vi "抓邊.vi"(0 "Image In":T1, 1 "Process":T7(ring), 2 "Optimized Mode":bool, 3 "Direction":T4(ring), 5 "ROI":T2, 9 "Gap":i32=10 min=1 max=300, 11 "error In":errorcluster, 12 "Edge Options":T5={"Edge Polarity"=0, "Kernel Size"=3, "Width"=3, "Minimum Edge Strength"=10.0, "Interpolation Type"=enum."Bilinear Fixed", "Data Processing Method"=enum."Average"} {"Edge Polarity" items=["All Edges", "Rising Edges", "Falling Edges"]; "Minimum Edge Strength" format="%.2f"; "Width" step=2; "Kernel Size" step=2}, 13 "Point Diameter (5)":u32=5 min=3 max=1000) -> (4 "Image Out":T1, 6 "Line Profile":T3(graph), 10 "Gradient Information":dbl[][](graph), 14 "Line Data":cluster{"X":sgl, "Y":sgl, "T":sgl}, 15 "error out":errorcluster)   [LabVIEW 2015]
uses:
  <vilib>/vision/Measure.llb/Edge Options.ctl
  <vilib>/vision/Measure.llb/Edge Polarity.ctl
  <vilib>/vision/Image Controls.llb/IMAQ Image.ctl
  <vilib>/vision/NI_Vision_Development_Module.lvlib
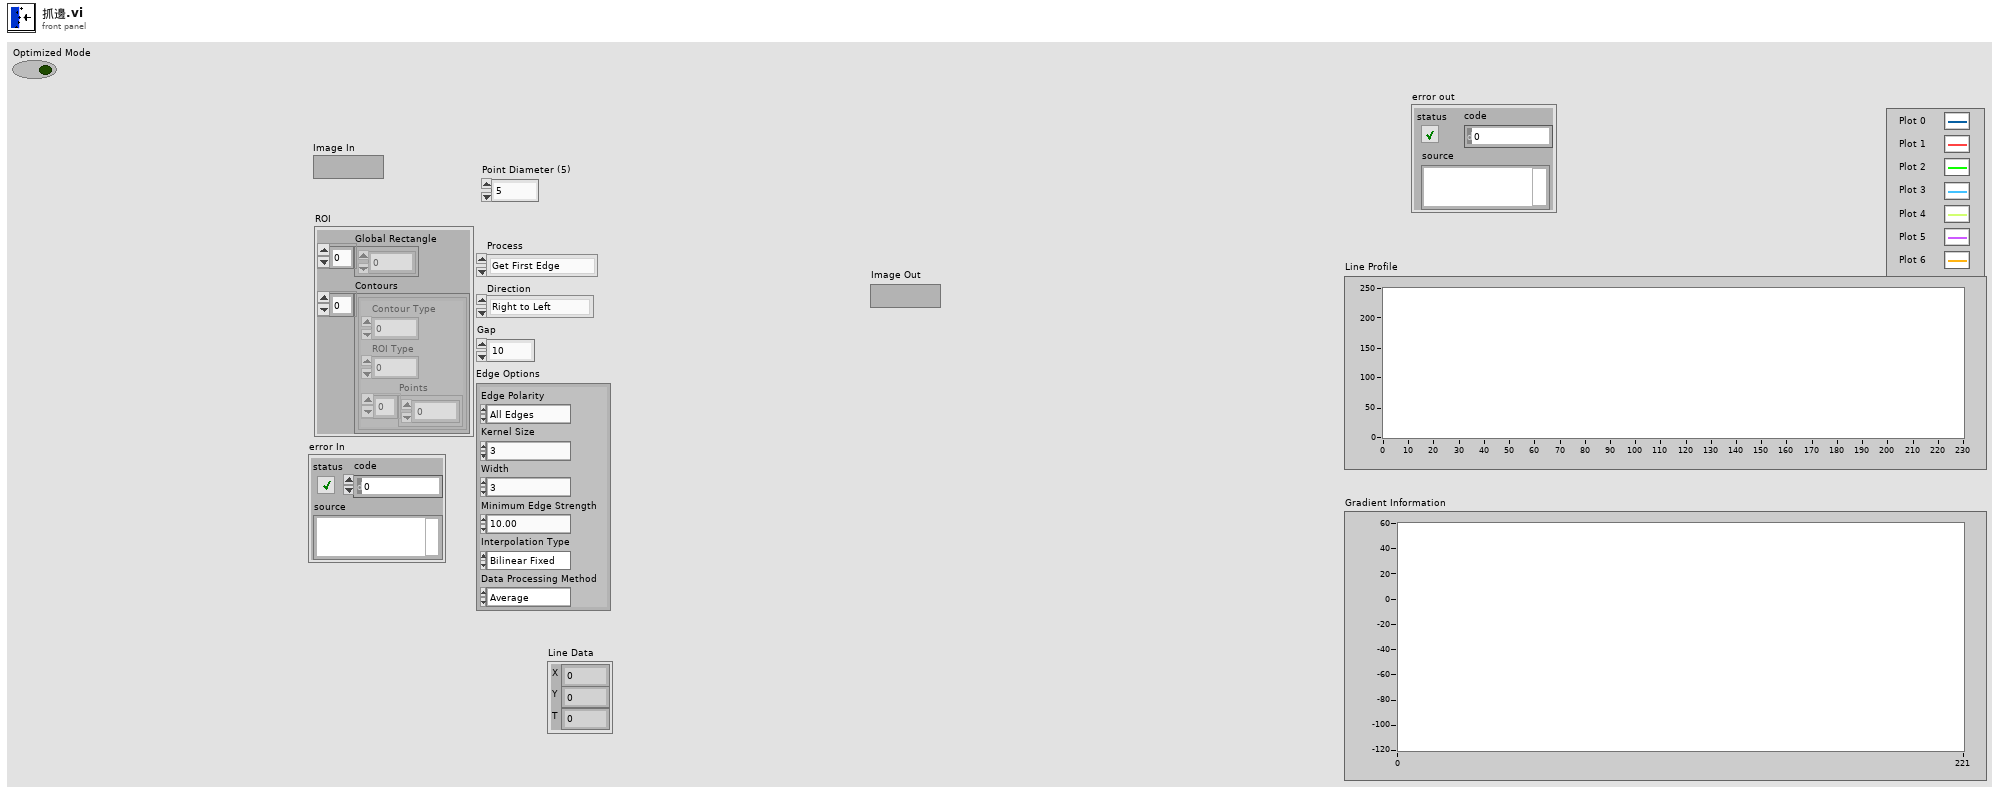
[diagram p1: front panel]
types:
  T1 = typedef "IMAQ Image.ctl" = refnum<image>
  T2 = cluster{"Global Rectangle":i32[], "Contours":cluster{"Contour Type":u32, "ROI Type":u32, "Points":i32[]}[]}
  T3 = cluster{"x0":sgl, "dx":sgl, "Pixels Line":sgl[]}[]
  T4 = enum16{"Right to Left", "Left  to Right", "Up to Down", "Down to Up"}
  T5 = typedef "Edge Options.ctl" = cluster{"Edge Polarity":T6, "Kernel Size":u32, "Width":u32, "Minimum Edge Strength":sgl, "Interpolation Type":enum32{"Zero Order", "Bilinear", "Quadratic", "Cubic", "Bilinear Fixed"}, "Data Processing Method":enum32{"Average", "Median"}}
  T6 = typedef "Edge Polarity.ctl" = u32
  T7 = enum16{"Get First Edge", "Get First + Last Edge", "Get All Edges", "Get Best Edge"}
  T8 = typedef "IMAQ Rectangle" = cluster{"Left":i32, "Top":i32, "Right":i32, "Bottom":i32, "Rotation":dbl}
  T9 = typedef "IMAQ Point" = cluster{"X":sgl, "Y":sgl}
  T10 = cluster{"Point 1":cluster{"x":dbl, "y":dbl}, "Point 2":cluster{"x":dbl, "y":dbl}}
  T11 = typedef "IMAQ Line" = cluster{"Start X":i32, "Start Y":i32, "End X":i32, "End Y":i32}
  T12 = typedef "ROI Descriptor" = cluster{"Global Rectangle":i32[], "Contours":cluster{"ID":enum32{"External", "Internal"}, "Type":u32, "Coordinates":i32[]}[]}
  T13 = typedef "Edge New.ctl" = cluster{"Location (Pixel)":cluster{"X":sgl, "Y":sgl}, "Location (Real-World)":cluster{"X":sgl, "Y":sgl}, "Distance (Pixel)":dbl, "Distance (Real-World)":dbl, "Strength":dbl, "Noise":dbl, "Rising?":bool}
  T14 = cluster{"Point 1":cluster{"X":sgl, "Y":sgl}, "Point 2":cluster{"X":sgl, "Y":sgl}}
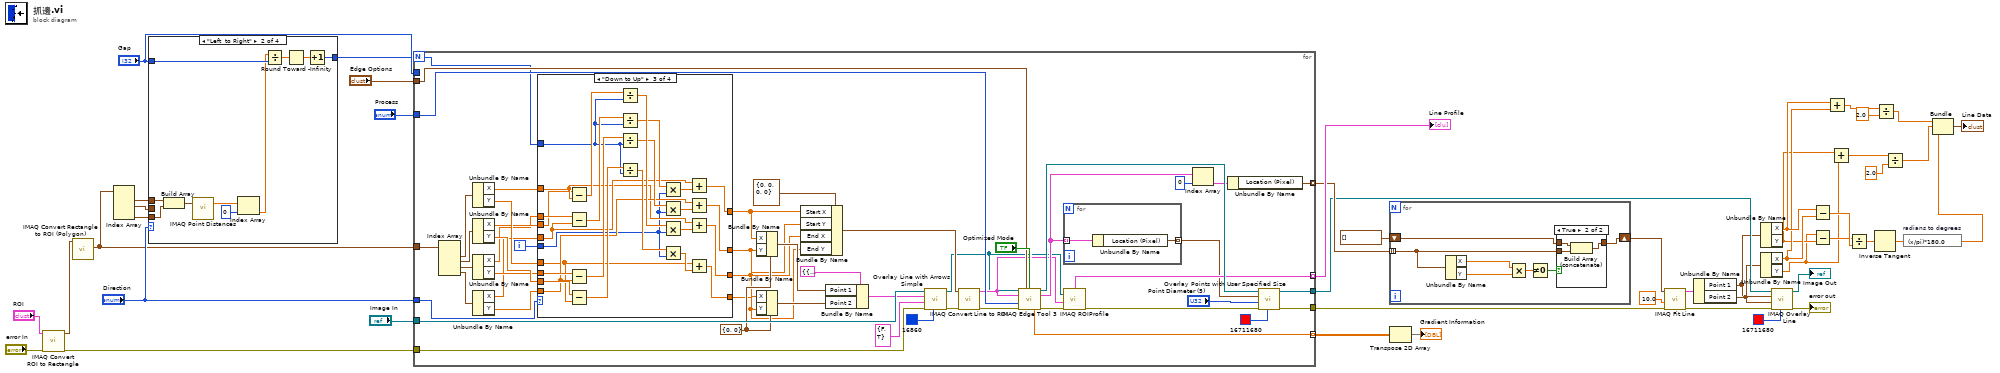
[diagram p0: block diagram]
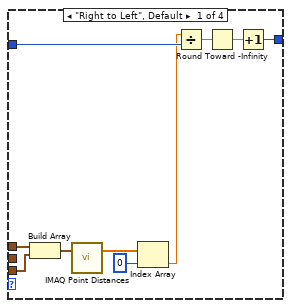
[diagram p2: hidden frame]
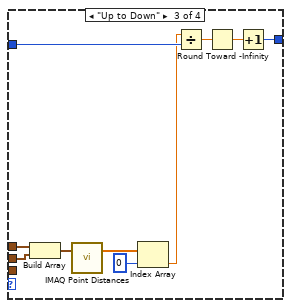
[diagram p3: hidden frame]
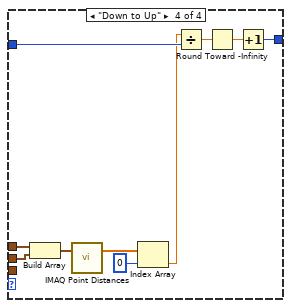
[diagram p4: hidden frame]
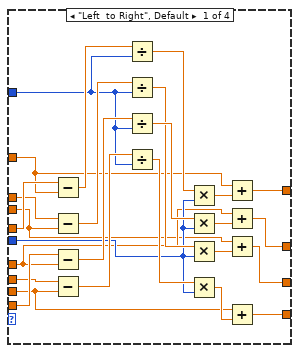
[diagram p6: hidden frame]
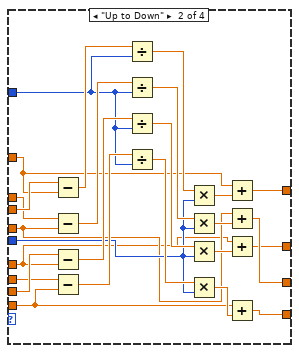
[diagram p7: hidden frame]
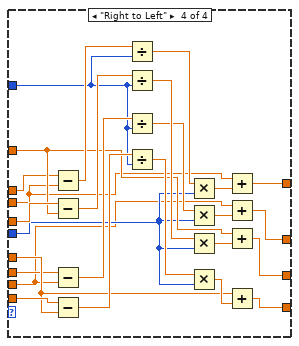
[diagram p8: hidden frame]
diagram:
  n1 = call "IMAQ Convert ROI to Rectangle"("error in (no error)"="error In", "ROI Descriptor"="ROI") -> ("error out"=w38:errorcluster, "Rectangle"=w26:T8)  [unwired: 7 in]
  n2 = call "IMAQ Convert Rectangle to ROI (Polygon)"("Rectangle"=w26) -> ("Rectangle Points"=w32:T9[])  [unwired: 7 in, 2 out]
  n3 = Index Array(array=w32) -> (element #1=w29:T9, element #2=w28:T9, element #4=w27:T9)  [unwired: 4 in, 1 out]
  n4 = case shown="\"Left  to Right\"" "Direction" {
    tunnel: "Gap" -> [w54 w64 w74 w84]
    tunnel: [w53 w63 w73 w83] -> w39
    tunnel: w29 -> [w50 w60 w72 w80]
    tunnel: w27 -> [w49 w59 _ _]
    tunnel: w28 -> [_ _ w68 w79]
    frame "Right to Left", Default {
      n5 = Build Array(w50, w49) -> (w52:T9[])
      n6 = call "IMAQ Point Distances"("Points"=w52) -> ("Distances"=w51:sgl[])  [unwired: 4 in, 1 out]
      n7 = Index Array(array=w51, index=0) -> (element=w47:sgl)
      n8 = Divide(x=w47, y=w54) -> (x/y=w55:sgl)
      n9 = Round Toward -Infinity(1:w55) -> (0:w56:sgl)
      n10 = Increment(x=w56) -> (x+1=w53:i32)
    }
    frame "Left  to Right" {
      n11 = Build Array(w60, w59) -> (w62:T9[])
      n12 = call "IMAQ Point Distances"("Points"=w62) -> ("Distances"=w61:sgl[])  [unwired: 4 in, 1 out]
      n13 = Index Array(array=w61, index=0) -> (element=w57:sgl)
      n14 = Divide(x=w57, y=w64) -> (x/y=w65:sgl)
      n15 = Round Toward -Infinity(1:w65) -> (0:w66:sgl)
      n16 = Increment(x=w66) -> (x+1=w63:i32)
    }
    frame "Up to Down" {
      n17 = Build Array(w72, w68) -> (w71:T9[])
      n18 = call "IMAQ Point Distances"("Points"=w71) -> ("Distances"=w70:sgl[])  [unwired: 4 in, 1 out]
      n19 = Index Array(array=w70, index=0) -> (element=w69:sgl)
      n20 = Divide(x=w69, y=w74) -> (x/y=w75:sgl)
      n21 = Round Toward -Infinity(1:w75) -> (0:w76:sgl)
      n22 = Increment(x=w76) -> (x+1=w73:i32)
    }
    frame "Down to Up" {
      n23 = Build Array(w80, w79) -> (w82:T9[])
      n24 = call "IMAQ Point Distances"("Points"=w82) -> ("Distances"=w81:sgl[])  [unwired: 4 in, 1 out]
      n25 = Index Array(array=w81, index=0) -> (element=w78:sgl)
      n26 = Divide(x=w78, y=w84) -> (x/y=w85:sgl)
      n27 = Round Toward -Infinity(1:w85) -> (0:w86:sgl)
      n28 = Increment(x=w86) -> (x+1=w83:i32)
    }
  }
  n29 = for {
    N: w39 -> [w124]
    tunnel: "Direction" -> [w122]
    tunnel: [w133] -> w35
    tunnel: "Image In" -> [w123]
    tunnel: w38 -> [w120]
    tunnel: [w132] -> w33
    tunnel: "Process" -> [w134]
    tunnel: "Edge Options" -> [w131]
    tunnel: [w130] -> w37 mode=indexing
    tunnel: [w129] -> w40 mode=indexing
    tunnel: [w128] -> w36 mode=indexing
    tunnel: "Gap" -> [_]
    tunnel: w32 -> [w119]
    i -> [w88]
    w116 = cluster{"X":i32, "Y":i32} {"X"=0, "Y"=0} ("Start Point")
    n30 = Index Array(array=w119) -> (element #1=w100:T9, element #2=w99:T9, element #3=w98:T9, element #4=w97:T9)  [unwired: 4 in]
    n31 = Unbundle By Name(w100) -> ("X"=w96:sgl, "Y"=w95:sgl)
    n32 = Unbundle By Name(w99) -> ("X"=w94:sgl, "Y"=w93:sgl)
    n33 = Unbundle By Name(w98) -> ("X"=w92:sgl, "Y"=w91:sgl)
    n34 = Unbundle By Name(w97) -> ("X"=w90:sgl, "Y"=w89:sgl)
    n35 = case shown="\"Down to Up\"" w122 {
      tunnel: [w149 w168 w194 w219] -> w108
      tunnel: [w144 w167 w193 w220] -> w105
      tunnel: [w147 w165 w191 w217] -> w107
      tunnel: [w143 w166 w192 w218] -> w106
      tunnel: w90 -> [w162 w173 w199 w229]
      tunnel: w96 -> [w140 w175 w198 w228]
      tunnel: w124 -> [w153 w177 w204 w230]
      tunnel: w88 -> [w152 w178 w195 w227]
      tunnel: w89 -> [w159 w169 w201 w224]
      tunnel: w95 -> [w142 w171 w200 w223]
      tunnel: w92 -> [w156 w174 w197 w226]
      tunnel: w94 -> [w141 w176 w196 w225]
      tunnel: w91 -> [w151 w170 w202 w222]
      tunnel: w93 -> [w139 w172 w203 w221]
      frame "Left  to Right", Default {
        n36 = Subtract(x=w162, y=w140) -> (x-y=w163:sgl)
        n37 = Subtract(x=w156, y=w141) -> (x-y=w158:sgl)
        n38 = Subtract(x=w159, y=w142) -> (x-y=w161:sgl)
        n39 = Subtract(x=w151, y=w139) -> (x-y=w154:sgl)
        n40 = Divide(x=w163, y=w153) -> (x/y=w164:sgl)
        n41 = Divide(x=w158, y=w153) -> (x/y=w157:sgl)
        n42 = Divide(x=w161, y=w153) -> (x/y=w160:sgl)
        n43 = Divide(x=w154, y=w153) -> (x/y=w155:sgl)
        n44 = Multiply(x=w164, y=w152) -> (x*y=w150:sgl)
        n45 = Multiply(x=w160, y=w152) -> (x*y=w148:sgl)
        n46 = Multiply(x=w157, y=w152) -> (x*y=w146:sgl)
        n47 = Multiply(x=w155, y=w152) -> (x*y=w145:sgl)
        n48 = Add(x=w140, y=w150) -> (x+y=w149:sgl)
        n49 = Add(x=w142, y=w148) -> (x+y=w147:sgl)
        n50 = Add(x=w141, y=w146) -> (x+y=w144:sgl)
        n51 = Add(x=w139, y=w145) -> (x+y=w143:sgl)
      }
      frame "Up to Down" {
        n52 = Subtract(x=w176, y=w175) -> (x-y=w189:sgl)
        n53 = Subtract(x=w174, y=w173) -> (x-y=w186:sgl)
        n54 = Subtract(x=w172, y=w171) -> (x-y=w188:sgl)
        n55 = Subtract(x=w170, y=w169) -> (x-y=w183:sgl)
        n56 = Divide(x=w189, y=w177) -> (x/y=w190:sgl)
        n57 = Divide(x=w186, y=w177) -> (x/y=w185:sgl)
        n58 = Divide(x=w188, y=w177) -> (x/y=w187:sgl)
        n59 = Divide(x=w183, y=w177) -> (x/y=w184:sgl)
        n60 = Multiply(x=w190, y=w178) -> (x*y=w182:sgl)
        n61 = Multiply(x=w185, y=w178) -> (x*y=w180:sgl)
        n62 = Multiply(x=w187, y=w178) -> (x*y=w181:sgl)
        n63 = Multiply(x=w184, y=w178) -> (x*y=w179:sgl)
        n64 = Add(x=w175, y=w182) -> (x+y=w168:sgl)
        n65 = Add(x=w173, y=w180) -> (x+y=w167:sgl)
        n66 = Add(x=w171, y=w181) -> (x+y=w165:sgl)
        n67 = Add(x=w169, y=w179) -> (x+y=w166:sgl)
      }
      frame "Down to Up" {
        n68 = Subtract(x=w196, y=w198) -> (x-y=w215:sgl)
        n69 = Subtract(x=w197, y=w199) -> (x-y=w212:sgl)
        n70 = Subtract(x=w202, y=w201) -> (x-y=w209:sgl)
        n71 = Subtract(x=w203, y=w200) -> (x-y=w214:sgl)
        n72 = Divide(x=w215, y=w204) -> (x/y=w216:sgl)
        n73 = Divide(x=w212, y=w204) -> (x/y=w211:sgl)
        n74 = Divide(x=w209, y=w204) -> (x/y=w210:sgl)
        n75 = Divide(x=w214, y=w204) -> (x/y=w213:sgl)
        n76 = Multiply(x=w211, y=w195) -> (x*y=w206:sgl)
        n77 = Multiply(x=w210, y=w195) -> (x*y=w205:sgl)
        n78 = Multiply(x=w216, y=w195) -> (x*y=w208:sgl)
        n79 = Multiply(x=w213, y=w195) -> (x*y=w207:sgl)
        n80 = Add(x=w199, y=w206) -> (x+y=w194:sgl)
        n81 = Add(x=w201, y=w205) -> (x+y=w191:sgl)
        n82 = Add(x=w198, y=w208) -> (x+y=w193:sgl)
        n83 = Add(x=w200, y=w207) -> (x+y=w192:sgl)
      }
      frame "Right to Left" {
        n84 = Subtract(x=w226, y=w225) -> (x-y=w238:sgl)
        n85 = Subtract(x=w229, y=w228) -> (x-y=w241:sgl)
        n86 = Subtract(x=w222, y=w221) -> (x-y=w235:sgl)
        n87 = Subtract(x=w224, y=w223) -> (x-y=w240:sgl)
        n88 = Divide(x=w238, y=w230) -> (x/y=w237:sgl)
        n89 = Divide(x=w241, y=w230) -> (x/y=w242:sgl)
        n90 = Divide(x=w235, y=w230) -> (x/y=w236:sgl)
        n91 = Divide(x=w240, y=w230) -> (x/y=w239:sgl)
        n92 = Multiply(x=w237, y=w227) -> (x*y=w232:sgl)
        n93 = Multiply(x=w236, y=w227) -> (x*y=w231:sgl)
        n94 = Multiply(x=w242, y=w227) -> (x*y=w234:sgl)
        n95 = Multiply(x=w239, y=w227) -> (x*y=w233:sgl)
        n96 = Add(x=w225, y=w232) -> (x+y=w219:sgl)
        n97 = Add(x=w221, y=w231) -> (x+y=w217:sgl)
        n98 = Add(x=w228, y=w234) -> (x+y=w220:sgl)
        n99 = Add(x=w223, y=w233) -> (x+y=w218:sgl)
      }
    }
    n100 = Bundle By Name(cluster=w116, "X"=w108, "Y"=w107) -> (w114:cluster{"X":i32, "Y":i32})
    n101 = Bundle By Name(cluster=w116, "X"=w105, "Y"=w106) -> (w115:cluster{"X":i32, "Y":i32})
    n102 = Bundle By Name(cluster=T11 {"Start X"=0, "Start Y"=0, "End X"=0, "End Y"=0} ("Line"), "Start X"=w108, "Start Y"=w107, "End X"=w105, "End Y"=w106) -> (w117:T11)
    n103 = Bundle By Name(cluster=T10 {"Point 1"={"x"=50.0, "y"=50.0}, "Point 2"={"x"=70.0, "y"=70.0}} ("Line Coordinates"), "Point 1"=w114, "Point 2"=w115) -> (w111:T10)
    n104 = call "Overlay Line with Arrows Simple.vi"("Color"=u32 16860, "error in"=w120, "Arrows"=cluster{"Start point":bool, "End point":bool} {"Start point"=FALSE, "End point"=TRUE}, "Line Coordinates"=w111, "Image In"=w123) -> ("error out"=w109:errorcluster, "Image Out"=w110:T1)  [unwired: 5 in]
    n105 = call "IMAQ Convert Line to ROI"("error in (no error)"=w109, "Line"=w117) -> ("error out"=w126:errorcluster, "ROI Descriptor"=w125:T12)  [unwired: 7 in]
    n106 = call "IMAQ Edge Tool 3"("Image"=w110, "Edge Options"=w131, "Optimized Mode"="Optimized Mode", "ROI Descriptor"=w125, "Process"=w134, "error in (no error)"=w126) -> ("Image (duplicate)"=w135:T1, "Edge Information"=w138:T13[], "Gradient Values"=w129:dbl[], "error out"=w127:errorcluster)  [unwired: 5 in, 1 out]
    n107 = for {
      tunnel: w138 -> [w244] mode=indexing
      tunnel: [w243] -> w101 mode=indexing
      n108 = Unbundle By Name(w244) -> ("Location (Pixel)"=w243:cluster{"X":sgl, "Y":sgl})
    }
    n109 = call "IMAQ ROIProfile"("error in (no error)"=w127, "ROI Descriptor"=w125, "Image"=w110) -> ("error out"=w137:errorcluster, "ROI Graph"=w130:cluster{"x0":sgl, "dx":sgl, "Pixels Line":sgl[]})  [unwired: 1 in, 3 out]
    n110 = Index Array(array=w138, index=0) -> (element=w102:T13)
    n111 = Unbundle By Name(w102) -> ("Location (Pixel)"=w128:cluster{"X":sgl, "Y":sgl})
    n112 = call "Overlay Points with User Specified Size.vi"("Color"=u32 16711680, "error in"=w137, "Point Diameter (5)"="Point Diameter (5)", "Points"=w101, "Image In"=w135) -> ("error out"=w132:errorcluster, "Image Out"=w133:T1)  [unwired: 5 in]
  }
  "Line Profile" <- w37
  n113 = for {
    tunnel: w36 -> [w247] mode=indexing
    shift-right: [w246] -> w34
    shift-left: cluster{"X":sgl, "Y":sgl}[] [] -> [w245]
    n114 = Unbundle By Name(w247) -> ("X"=w251:sgl, "Y"=w250:sgl)
    n115 = Multiply(x=w251, y=w250) -> (x*y=w249:sgl)
    n116 = Not Equal To 0?(x=w249) -> (x != 0?=w248:bool)
    n117 = case shown="True" w248 {
      tunnel: w247 -> [_ w255]
      tunnel: [w252 w254] -> w246
      tunnel: w245 -> [w252 w253]
      frame False {
      }
      frame True {
        n118 = Build Array (concatenate)(w253, w255) -> (w254:cluster{"X":sgl, "Y":sgl}[])
      }
    }
  }
  n119 = Transpose 2D Array(2D array=w40) -> (transposed array=→"Gradient Information":dbl[][])
  n120 = call "IMAQ Fit Line"("error in (no error)"=w33, "Pixel Radius"=sgl 10.0, "Points"=w34) -> ("error out"=w17:errorcluster, "Line Segment"=w15:T14)  [unwired: 3 in, 4 out]
  n121 = Unbundle By Name(w15) -> ("Point 1"=w18:cluster{"X":sgl, "Y":sgl}, "Point 2"=w19:cluster{"X":sgl, "Y":sgl})
  n122 = Unbundle By Name(w18) -> ("X"=w12:sgl, "Y"=w10:sgl)
  n123 = Unbundle By Name(w19) -> ("X"=w11:sgl, "Y"=w9:sgl)
  n124 = call "IMAQ Overlay Line"("Color"=u32 16711680, "error in (no error)"=w17, "End Point"=w19, "Start Point"=w18, "Image"=w35) -> ("error out"=→"error out":errorcluster, "Image Out"=→"Image Out":T1)  [unwired: 5 in]
  n125 = Subtract(x=w12, y=w11) -> (x-y=w23:sgl)
  n126 = Subtract(x=w9, y=w10) -> (x-y=w22:sgl)
  n127 = Add(x=w12, y=w11) -> (x+y=w7:sgl)
  n128 = Add(x=w10, y=w9) -> (x+y=w8:sgl)
  n129 = Divide(x=w22, y=w23) -> (x/y=w21:sgl)
  n130 = Inverse Tangent(1:w21) -> (0:w20:sgl)
  n131 = Divide(x=w7, y=sgl 2.0) -> (x/y=w4:sgl)
  n132 = Divide(x=w8, y=sgl 2.0) -> (x/y=w3:sgl)
  n133 = expression code="(x/pi)*180.0" "radians to degrees"(w20) -> (w2:sgl)
  n134 = Bundle(w4, w3, w2) -> (→"Line Data":cluster{sgl, sgl, sgl})  [unwired: 1 in]
